vi "FF_move_address_back_to_default.vi"() -> ()   [LabVIEW 2010]
panel:
  in  "link name":string="interface0-0"
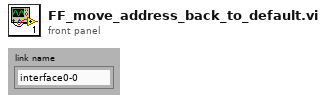
[diagram p1: front panel]
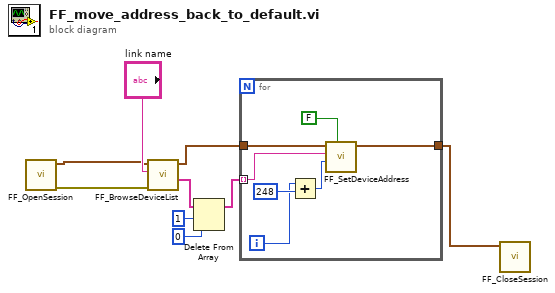
[diagram p0: block diagram]
diagram:
  n1 = call "FF_OpenSession.vi"() -> ("error out"=w7:errorcluster, "refnum out"=w8:cluster{"Handle1":u32, "Handle2":u32})  [unwired: 10 in]
  n2 = call "FF_BrowseDeviceList.vi"("error in (no error)"=w7, "link name"="link name", "refnum in"=w8) -> ("deviceID list"=w4:string[], "refnum out"=w6:cluster{"Handle1":u32, "Handle2":u32})  [unwired: 4 in, 3 out]
  n3 = Delete From Array(array=w4, length=1, index=0) -> (array with subset deleted=w3:string[])  [unwired: 1 out]
  n4 = for {
    tunnel: w3 -> [w16] mode=indexing
    tunnel: w6 -> [w15]
    tunnel: [w10] -> w5
    i -> [w12]
    n5 = Add(x=w12, y=248) -> (x+y=w11:i32)
    n6 = call "FF_SetDeviceAddress.vi"("Is pdTag"=FALSE, "address"=w11, "pdTag/deviceID"=w16, "refnum in"=w15) -> ("refnum out"=w10:cluster{"Handle1":u32, "Handle2":u32})  [unwired: 6 in, 1 out]
  }
  n7 = call "FF_CloseSession.vi"("refnum in"=w5) -> ()  [unwired: 10 in, 1 out]
